vi "ArraySize.vi"() -> ()   [LabVIEW 2021]
panel:
  out "size(s)":i32
  in  "Array":dbl[](array[numeric])
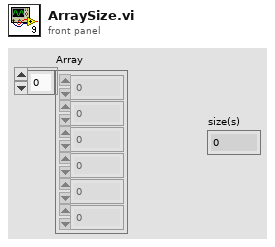
[diagram p1: front panel]
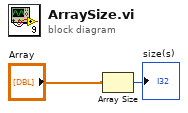
[diagram p0: block diagram]
diagram:
  n1 = Array Size(array="Array") -> (size(s)=→"size(s)":i32)
